vi "RunTestforUSB.vi"(5 "Attenuation":u32, 7 "Dwell Time (s)":dbl, 8 "error in":errorcluster, 9 "End Frequency (khz)":u32, 10 "Start Frequency (khz)":u32, 11 "VISA resource name":refnum<visa-resource-name>) -> (0 "error out":errorcluster, 2 "Log":string)   [LabVIEW 2013]
uses:
  <vilib>/Instr/_visa.llb/VISA Configure Serial Port (Instr).vi
panel:
  in  "stop":bool
  in  "Start Test":bool
  in  "Timings":i32[](array[numeric])=[40, 40, 40, 40, 1000, 40]
  out "start":dbl format="%_19f"
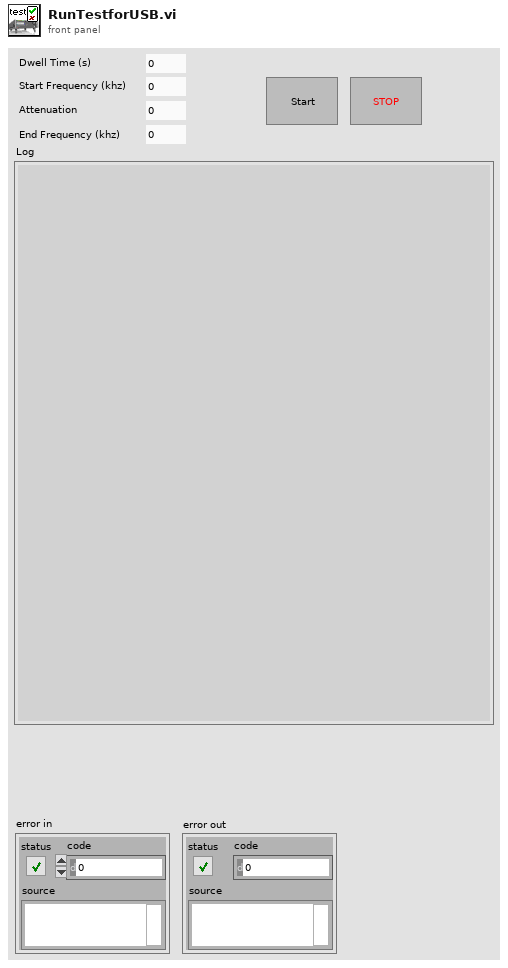
[diagram p1: front panel]
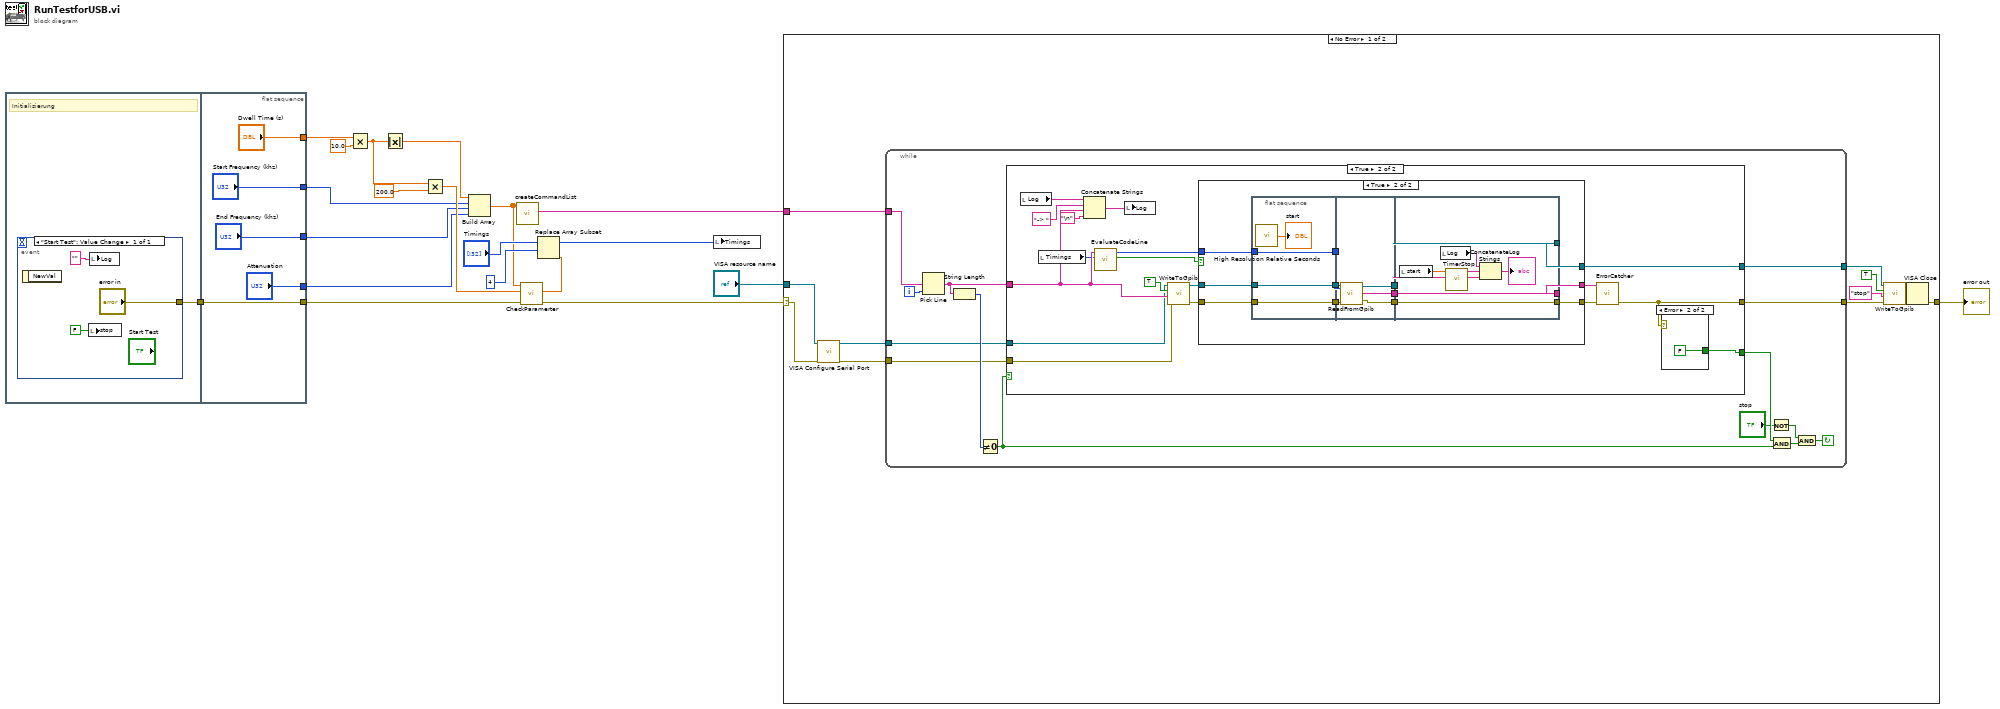
[diagram p0: block diagram]
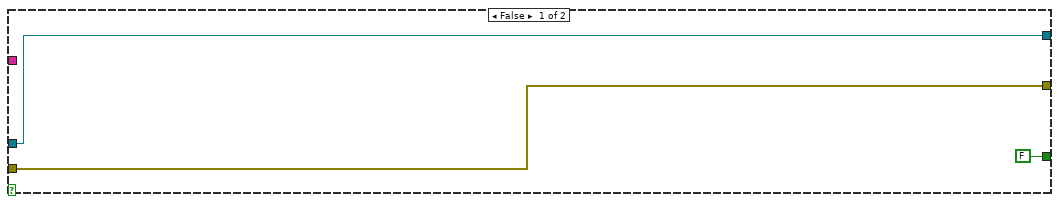
[diagram p2: hidden frame]
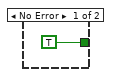
[diagram p3: hidden frame]
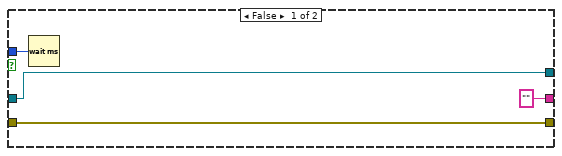
[diagram p4: hidden frame]
diagram:
  n1 = flat-sequence {
    tunnel: [w20] -> w8
    tunnel: [w28] -> w9
    tunnel: w8 -> [w28]
    tunnel: ["Dwell Time (s)"] -> w6
    tunnel: ["Attenuation"] -> w7
    tunnel: ["End Frequency (khz)"] -> w1
    tunnel: ["Start Frequency (khz)"] -> w2
    frame #0 {
      # "Initialisierung"
      n2 = event shown="[0] \"Start Test\": Value Change" {
        selector: _ -> [_]
        dyn-events: _ -> [_]
        timeout: _ -> [_]
        tunnel: ["error in"] -> w20
        event "Start Test": Value Change {
          n3 = event-data() -> ()  [unwired: 1 in, 1 out]
          n4 = local write "stop"(FALSE) -> ()
          n5 = local write "Log"("") -> ()
        }
      }
    }
    frame #1 {
    }
  }
  n6 = Multiply(x=w6, y=10.0) -> (x*y=w4:dbl)
  n7 = Absolute Value(x=w4) -> (abs(x)=w3:dbl)
  n8 = Multiply(x=w4, y=200.0) -> (x*y=w13:dbl)
  n9 = Build Array(w3, w2, w1, w7) -> (w10:dbl[])
  n10 = call "createCommandList.vi"("Array"=w10) -> ("String"=w18:string)  [unwired: 9 in]
  n11 = call "CheckParamerter.vi"("error in (no error)"=w9, "Array"=w10) -> ("error out"=w11:errorcluster)  [unwired: 9 in]
  n12 = Replace Array Subset(array="Timings", new element=w13, index=4) -> (w17:i32[])
  n13 = local write "Timings"(w17) -> ()
  n14 = case shown="No Error" w11 {
    selector: w11 -> [w31 w111]
    tunnel: "VISA resource name" -> [w32 _]
    tunnel: w18 -> [w40 _]
    tunnel: [w39 w111] -> w12
    frame No Error {
      n15 = call-poly "VISA Configure Serial Port"("VISA resource name"=w32, "error in (no error)"=w31) -> ("VISA resource name out"=w30:refnum<visa-resource-name>, "error out"=w29:errorcluster)  [unwired: 12 in]
      n16 = while {
        tunnel: [w53] -> w35
        tunnel: [w52] -> w36
        tunnel: w40 -> [w49]
        tunnel: w30 -> [w42]
        tunnel: w29 -> [w41]
        i -> [w54]
        stop <- w43 continue-if-true
        n17 = Pick Line(multi-line string=w49, line index=w54) -> (output string=w51:string)  [unwired: 1 in]
        n18 = String Length(string=w51) -> (length=w50:i32)
        n19 = Not Equal To 0?(x=w50) -> (x != 0?=w47:bool)
        n20 = case shown="True" w47 {
          tunnel: [w55 w60] -> w53
          tunnel: [w56 w61] -> w52
          tunnel: w51 -> [_ w73]
          tunnel: [FALSE w63] -> w48
          tunnel: w42 -> [w56 w59]
          tunnel: w41 -> [w55 w58]
          frame False {
          }
          frame True {
            n21 = local read "Log"() -> (w66:string)
            n22 = local read "Timings"() -> (w62:i32[])
            n23 = Concatenate Strings(w66, "-> " ("string"), w73, "\n") -> (w69:string)
            n24 = call "EvaluateCodeLine.vi"("Timings"=w62, "input string"=w73) -> ("read"=w74:bool, "timeout (ms)"=w75:i32)  [unwired: 8 in]
            n25 = local write "Log"(w69) -> ()
            n26 = call "WriteToGpib.vi"("error in (no error)"=w58, "String to Send"=w73, "checksum"=TRUE, "VISA Refnum in"=w59) -> ("error out"=w71:errorcluster, "VISA Refnum out"=w72:refnum<visa-resource-name>)  [unwired: 6 in]
            n27 = case shown="True" w74 {
              tunnel: [w80 w93] -> w61
              tunnel: w75 -> [w81 w91]
              tunnel: [w79 w92] -> w65
              tunnel: ["" ("Return String") w88] -> w64
              tunnel: w72 -> [w80 w90]
              tunnel: w71 -> [w79 w89]
              frame False {
                n28 = Wait (ms)(milliseconds to wait=w81) -> ()  [unwired: 1 out]
              }
              frame True {
                n29 = flat-sequence {
                  tunnel: w89 -> [w96]
                  tunnel: w90 -> [w97]
                  tunnel: w91 -> [w94]
                  tunnel: [w94] -> w84
                  tunnel: [w97] -> w83
                  tunnel: [w96] -> w82
                  tunnel: [w103] -> w87
                  tunnel: [w102] -> w86
                  tunnel: [w101] -> w85
                  tunnel: w84 -> [w98]
                  tunnel: w83 -> [w100]
                  tunnel: w82 -> [w99]
                  tunnel: [w107] -> w88
                  tunnel: [w109] -> w92
                  tunnel: [w110] -> w93
                  tunnel: w87 -> [w110]
                  tunnel: w86 -> [w109]
                  tunnel: w85 -> [w107]
                  frame #0 {
                    n30 = call <vilib>:"High Resolution Relative Seconds.vi"() -> ("relative seconds"=→"start":dbl)
                  }
                  frame #1 {
                    n31 = call "ReadFromGpib.vi"("COM Port"=w100, "timeout (ms)"=w98, "Error in"=w99) -> ("VISA resource name out"=w103:refnum<visa-resource-name>, "Return String"=w101:string, "Error Out"=w102:errorcluster)  [unwired: 3 in]
                  }
                  frame #2 {
                    n32 = local read "start"() -> (w108:dbl)
                    n33 = local read "Log"() -> (w105:string)
                    n34 = call "TimerStop.vi"("Start Zeit"=w108) -> ("String"=w104:string)  [unwired: 10 in]
                    n35 = Concatenate Strings(w105, w104, w107) -> (→"Log":string)
                  }
                }
              }
            }
            n36 = call "ErrorCatcher.vi"("error in"=w65, "input String"=w64) -> ("error out"=w60:errorcluster)  [unwired: 9 in]
            n37 = case shown="Error" w60 {
              tunnel: [TRUE FALSE] -> w63
              frame No Error {
              }
              frame Error {
              }
            }
          }
        }
        n38 = Not(x="stop") -> (.not. x?=w44:bool)
        n39 = And(x=w48, y=w47) -> (x .and. y?=w46:bool)
        n40 = And(x=w44, y=w46) -> (x .and. y?=w43:bool)
      }
      n41 = call "WriteToGpib.vi"("error in (no error)"=w35, "String to Send"="stop", "checksum"=TRUE, "VISA Refnum in"=w36) -> ("error out"=w33:errorcluster, "VISA Refnum out"=w34:refnum<visa-resource-name>)  [unwired: 6 in]
      n42 = VISA Close(VISA resource name=w34, error in (no error)=w33) -> (error out=w39:errorcluster)
    }
    frame Error {
    }
  }
  "error out" <- w12
